vi "Builder-Get Build Info.vi"(0 "Project Path in":path, 7 "Project Item":refnum<vi>, 11 "error in (no error)":errorcluster) -> (4 "Project Path out":path, 6 "Build Spec Name":string, 8 "Exe Path":path, 10 "Product Name":string, 15 "error out":errorcluster)   [LabVIEW 2020]
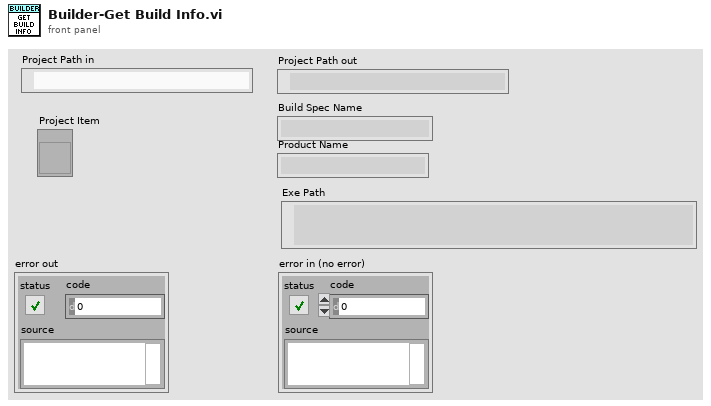
[diagram p1: front panel]
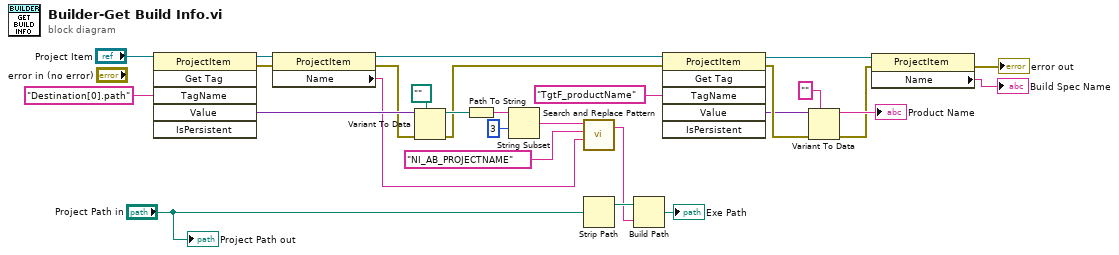
[diagram p0: block diagram]
diagram:
  n1 = invoke class="ProjectItem" method="Get Tag"(reference="Project Item", "TagName"="Destination[0].path" ("Tag Name")) -> (reference out=w4:refnum<vi>, error out=w2:errorcluster, "Value"=w21:variant)  [unwired: 4 in, 3 out]
  n2 = property class="ProjectItem"(reference=w4, error in=w2) -> (reference out=w3:refnum<vi>, error out=w1:errorcluster, "Name"=w5:string)
  n3 = Variant To Data(error in=w1, type=path "" ("appended path"), Variant=w21) -> (data=w18:path, error out=w14:errorcluster)
  n4 = Path To String(path=w18) -> (string=w17:string)
  n5 = String Subset(string=w17, offset (0)=3) -> (substring=w8:string)  [unwired: 1 in]
  n6 = call <vilib>:"Search and Replace Pattern.vi"("string"=w8, "regular expression (\"\")"="NI_AB_PROJECTNAME" ("regular expression (\"\")"), "replace string (\"\")"=w5) -> ("result string"=w9:string)  [unwired: 2 in, 1 out]
  n7 = Strip Path(path="Project Path in") -> (stripped path=w22:path)  [unwired: 1 out]
  n8 = Build Path(base path=w22, name or relative path=w9) -> (appended path=→"Exe Path":path)
  n9 = invoke class="ProjectItem" method="Get Tag"(reference=w3, error in=w14, "TagName"="TgtF_productName" ("Tag Name")) -> (reference out=w13:refnum<vi>, error out=w26:errorcluster, "Value"=w25:variant)  [unwired: 3 in, 3 out]
  n10 = Variant To Data(error in=w26, type="", Variant=w25) -> (data=→"Product Name":string, error out=w12:errorcluster)
  n11 = property class="ProjectItem"(reference=w13, error in=w12) -> (error out=→"error out":errorcluster, "Name"=→"Build Spec Name":string)  [unwired: 1 out]
  "Project Path out" <- "Project Path in"
